vi "TDS Digital Output Write.vi"(8 "error in (no error)":errorcluster, 9 "State":bool, 10 "Signal InstConfig":string, 11 "Address":string) -> (0 "error out":errorcluster)   [LabVIEW 2025, in "Interface Functions.lvlib"]
uses:
  Interface Functions.lvlib
panel:
  # "Digital Output Write"
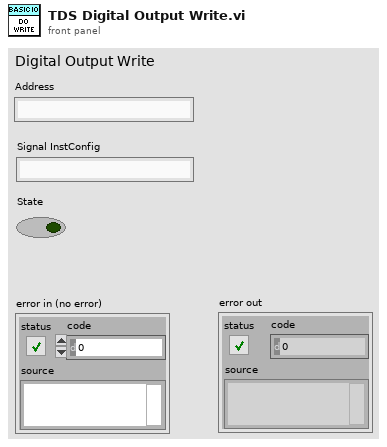
[diagram p1: front panel]
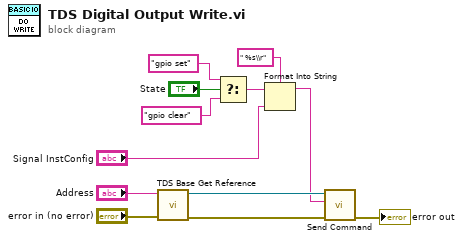
[diagram p0: block diagram]
diagram:
  n1 = call "TDS Base Get Reference.vi"("error in (no error)"="error in (no error)", "Address"="Address") -> ("error out"=w4:errorcluster, "Reference"=w3:refnum<visa-resource-name>)  [unwired: 8 in]
  n2 = Select(t="gpio set", s="State", f="gpio clear") -> (s? t:f=w8:string)
  n3 = Format Into String(format string=" %s\\r", initial string=w8, "Signal InstConfig") -> (resulting string=w2:string)  [unwired: 1 in, 1 out]
  n4 = call "Send Command.vi"("error in (no error)"=w4, "Command"=w2, "VISA resource name"=w3) -> ("error out"=→"error out":errorcluster)  [unwired: 6 in, 2 out]
